vi "Read_Write_Trav_Config.vi"(1 "Traverse Name":string, 2 "Mode":T1(ring)) -> (0 "Error String":string)   [LabVIEW 2022 SP3]
uses:
  Anemometry/Anemometry Sub Vis/Globals/Constants_global.vi
  DriveConfigGlobal.vi
  Anemometry/Anemometry Sub Vis/Globals/Trav_pos_global.vi
  Serial Link Layer/subVIs/Serial_Logging_Global.vi
  <vilib>/Instr/_visa.llb/VISA Find Search Mode.ctl
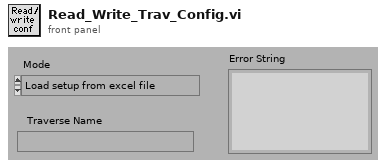
[diagram p1: front panel]
types:
  T1 = enum16{"Load setup from excel file", "Save setup to excel file"}
  T2 = typedef "DriveProperties.ctl" = cluster{"Channel Name":string, "Vel. Default":sgl, "Acc. Default":sgl, "Vel. Max":sgl, "Vel. Min":sgl, "Acc. Max":sgl, "Acc. Min":sgl, "Pulses/unit":sgl, "Address":u8, "Pulse Offset":i32, "Pos Tolerance":sgl, "Pulses/rev":sgl, "Backlash/Eng units":sgl, "Current Pos":sgl, "Ch Status":enum16{"Active", "Offline", "Simulate"}, "Port Name":string, "Axis Transform mode":string, "Metadata Ch Name":string, "Type":string, "De Power Motor":enum16{"TRUE", "FALSE"}, "ConfigString":string}
  T3 = typedef "VISA Find Search Mode.ctl" = u32
  T4 = typedef "Port_Params.ctl" = cluster{"Name":string, "flow control etc.":cluster{"input XON/XOFF":bool, "input HW Handshake":bool, "input alt HW HShk":bool, "output XON/XOFF":bool, "output HW Handshake":bool, "output alt HW HShk":bool, "XOFF byte ":u8, "XON byte":u8, "parity err byte":u16}, "buffer size":u16, "baud rate":u32, "data bits":u16, "stop bits":enum16{"1 bit", "1.5 bits", "2 bits"}, "parity":enum16{"no parity", "odd parity", "even parity", "mark parity", "space parity"}}
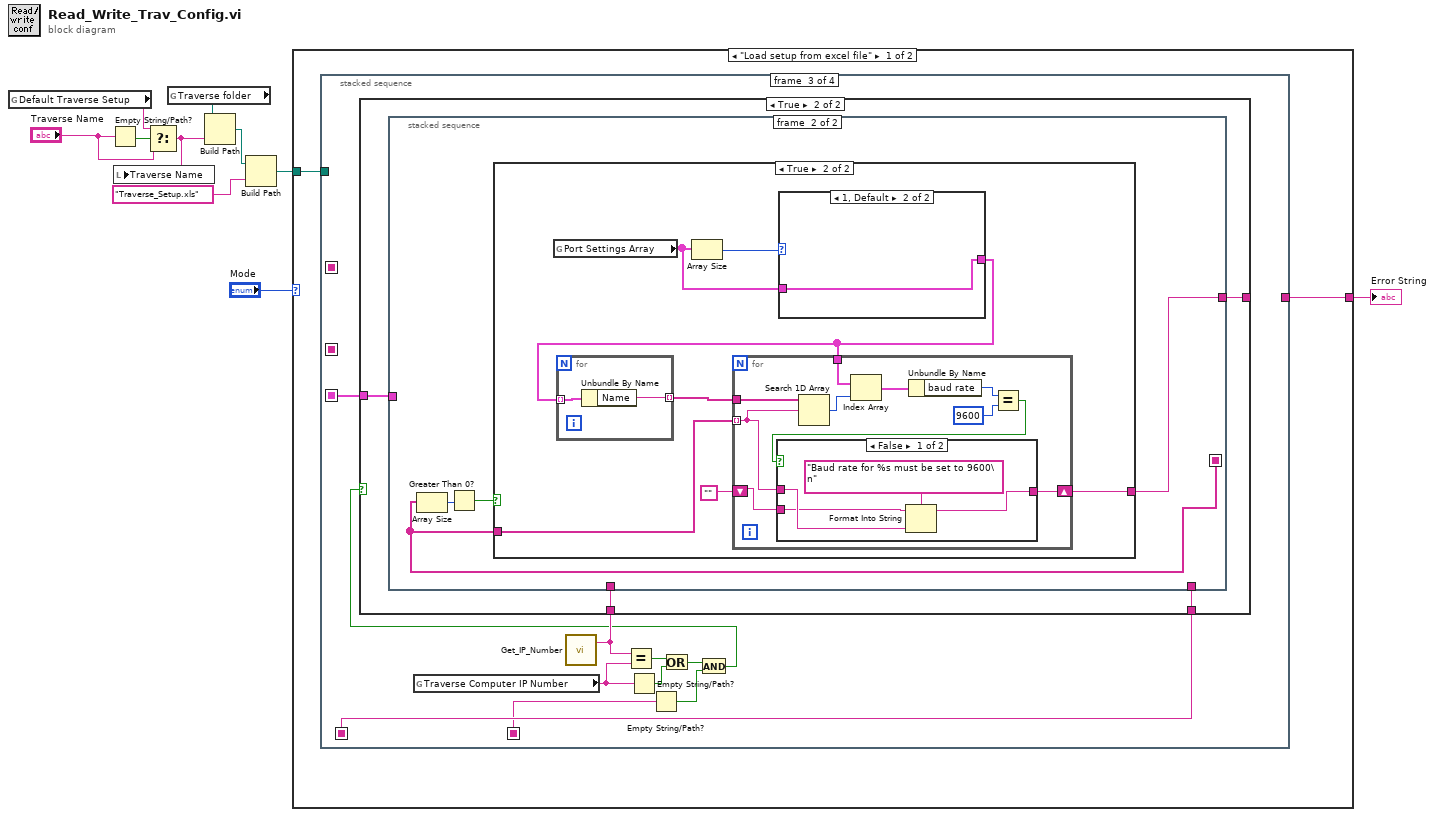
[diagram p0: block diagram]
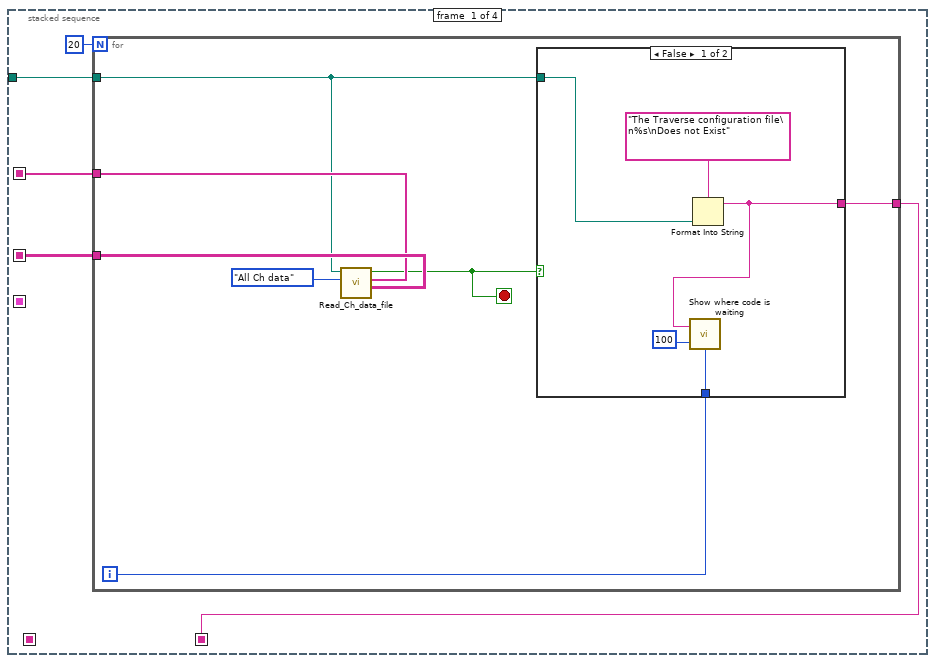
[diagram p2: hidden frame]
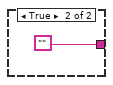
[diagram p3: hidden frame]
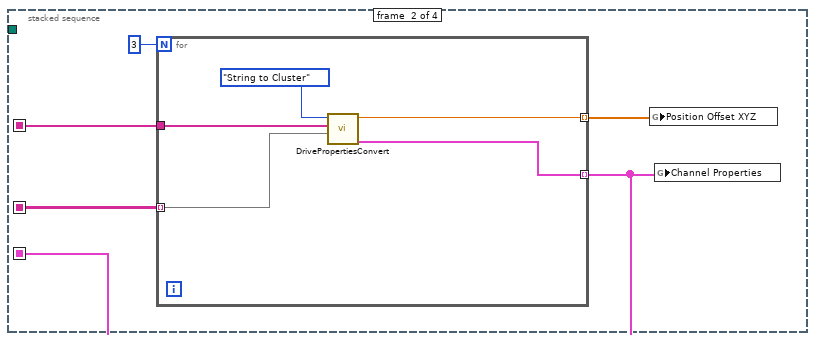
[diagram p4: hidden frame]
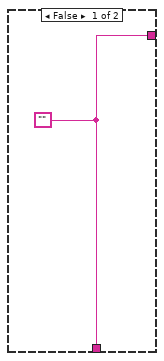
[diagram p5: hidden frame]
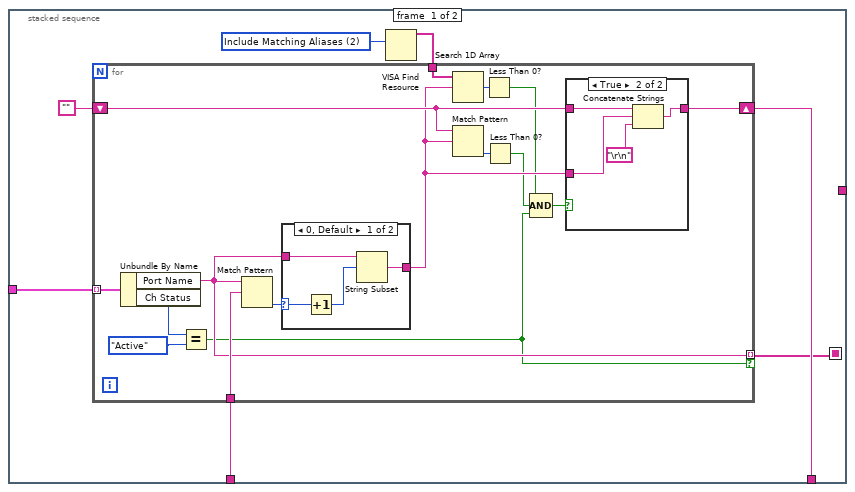
[diagram p6: hidden frame]
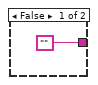
[diagram p9: hidden frame]
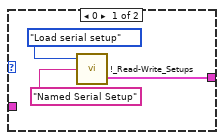
[diagram p11: hidden frame]
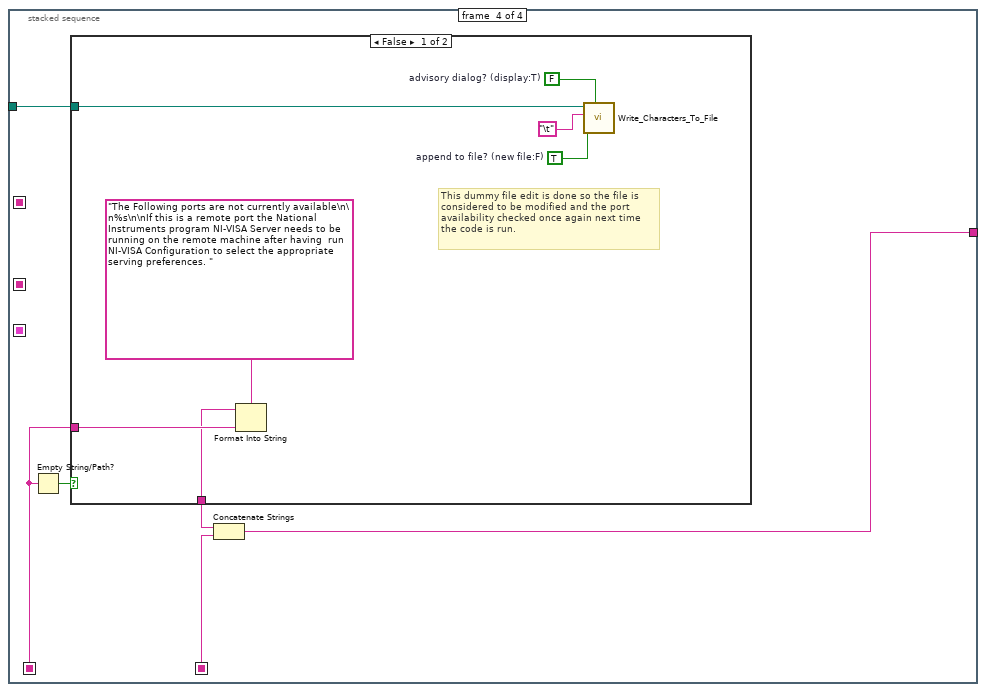
[diagram p12: hidden frame]
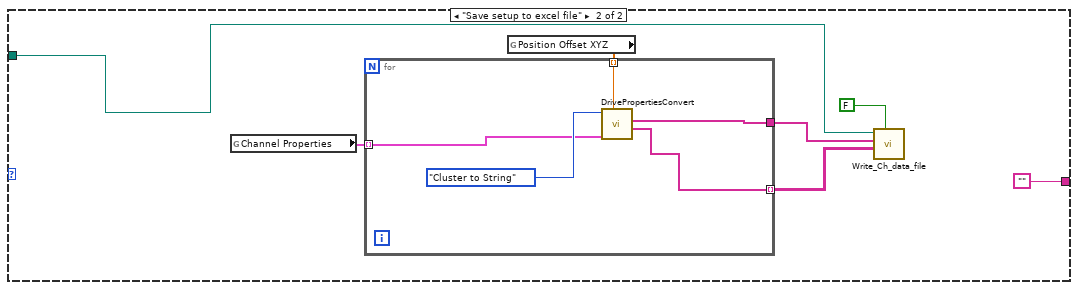
[diagram p14: hidden frame]
diagram:
  n1 = global read "Trav_pos_global.vi" "Default Traverse Setup"() -> (w5:string)
  n2 = Empty String/Path?(string/path="Traverse Name") -> (empty?=w6:bool)
  n3 = Select(t=w5, s=w6, f="Traverse Name") -> (s? t:f=w2:string)
  n4 = local write "Traverse Name"(w2) -> ()
  n5 = global read "Constants_global.vi" "Traverse folder"() -> (w8:path)
  n6 = Build Path(base path=w8, name or relative path=w2) -> (appended path=w7:path)
  n7 = Build Path(base path=w7, name or relative path="Traverse_Setup.xls" ("Substring")) -> (appended path=w9:path)
  n8 = case shown="\"Load setup from excel file\"" "Mode" {
    tunnel: w9 -> [w12 w142]
    tunnel: [w11 ""] -> w1
    frame "Load setup from excel file" {
      n9 = stacked-sequence {
        seq-local: [w17 _ _ _] -> [_ w34 _ _]
        seq-local: [w16 _ _ _] -> [_ w35 _ _]
        seq-local: [_ w33 _ _] -> [_ _ w50 _]
        seq-local: [_ _ w49 _] -> [_ _ _ w126]
        seq-local: [w13 _ _ _] -> [_ _ w41 w123]
        tunnel: w12 -> [w15 _ _ w125]
        tunnel: [_ _ _ w122] -> w11
        frame #0 {
          n10 = for {
            N: 20 -> [_]
            tunnel: [w23] -> w17
            tunnel: [w22] -> w16
            tunnel: w15 -> [w21]
            tunnel: [w20] -> w13
            i -> [w18]
            stop <- w19 stop-if-true
            n11 = call "Read_Ch_data_file.vi"("Output"=enum16{"All Ch data", "The last few rows"}."All Ch data", "Filename"=w21) -> ("Channel Values"=w23:string[][], "Merged Channels"=w22:string[], "exists?"=w19:bool)  [unwired: 3 in, 2 out]
            n12 = case shown="False" w19 {
              tunnel: w21 -> [w29 _]
              tunnel: [w26 ""] -> w20
              tunnel: w18 -> [w25 _]
              frame False {
                n13 = Format Into String(format string="The Traverse configuration file\n%s\nDoes not Exist" ("Format String"), w29) -> (resulting string=w26:string)  [unwired: 2 in, 1 out]
                n14 = call "Show where code is waiting.vi"("Loop index"=w25, "Wait (ms)"=u32 100 ("milliseconds to wait"), "Message"=w26) -> ()  [unwired: 1 in]
              }
              frame True {
              }
            }
          }
        }
        frame #1 {
          n15 = for {
            N: 3 -> [_]
            tunnel: w35 -> [w39]
            tunnel: w34 -> [w38] mode=indexing
            tunnel: [w36] -> w33 mode=indexing
            tunnel: [w37] -> w32 mode=indexing
            n16 = call "DrivePropertiesConvert.vi"("String in"=w38, "Ch names In"=w39, "Mode"=enum16{"Cluster to String", "String to Cluster"}."String to Cluster") -> ("Channel Properties Out"=w36:T2, "Position Offset Out"=w37:dbl)  [unwired: 2 in, 2 out]
          }
          n17 = global write "DriveConfigGlobal.vi" "Position Offset XYZ"(w32) -> ()
          n18 = global write "DriveConfigGlobal.vi" "Channel Properties"(w33) -> ()
        }
        frame #2 {
          n19 = global read "Trav_pos_global.vi" "Traverse Computer IP Number"() -> (w47:string)
          n20 = call "Get_IP_Number.vi"() -> ("IP Number"=w48:string)  [unwired: 1 out]
          n21 = Equal?(x=w48, y=w47) -> (x = y?=w45:bool)
          n22 = Empty String/Path?(string/path=w47) -> (empty?=w46:bool)
          n23 = Empty String/Path?(string/path=w41) -> (empty?=w44:bool)
          n24 = Or(x=w45, y=w46) -> (x .or. y?=w43:bool)
          n25 = And(x=w43, y=w44) -> (x .and. y?=w42:bool)
          n26 = case shown="True" w42 {
            tunnel: w50 -> [_ w55]
            tunnel: [w51 w54] -> w49
            tunnel: w48 -> [_ w53]
            tunnel: [w51 w52] -> _
            frame False {
              w51 = ""
            }
            frame True {
              n27 = stacked-sequence {
                seq-local: [w57 _] -> [_ w90]
                tunnel: w55 -> [w62 _]
                tunnel: [w59 _] -> w54
                tunnel: w53 -> [w58 _]
                tunnel: [_ w89] -> w52
                frame #0 {
                  w56 = T3 2 items=["Canonical Names Only"=0, "Aliases Only"=1, "Include Matching Aliases"=2, "Include All Aliases"=4] ("Search Mode")
                  n28 = VISA Find Resource(10:w56) -> (3:w61:string[])  [unwired: 1 in, 3 out]
                  n29 = for {
                    tunnel: w58 -> [w78]
                    tunnel: w62 -> [w76] mode=indexing
                    tunnel: w61 -> [w75]
                    shift-right: [w74] -> w59
                    shift-left: "" -> [w73]
                    tunnel: [w66] -> w57 mode=indexing if=w65
                    n30 = Unbundle By Name(w76) -> ("Port Name"=w66:string, "Ch Status"=w64:enum16{"Active", "Offline", "Simulate"})
                    n31 = Equal?(x=w64, y=enum16{"Active", "Offline", "Simulate"}."Active" ("Channel Properties.Ch Status")) -> (x = y?=w65:bool)
                    n32 = Match Pattern(string=w66, regular expression=w78) -> (offset past match=w77:i32)  [unwired: 4 out]
                    n33 = case shown="0, Default" w77 {
                      selector: w77 -> [w84 _]
                      tunnel: [w85 w88] -> w72
                      tunnel: w66 -> [w86 w88]
                      frame 0, Default {
                        n34 = Increment(x=w84) -> (x+1=w87:i32)
                        n35 = String Subset(string=w86, offset (0)=w87) -> (substring=w85:string)  [unwired: 1 out]
                      }
                      frame -1 {
                      }
                    }
                    n36 = Search 1D Array(1D array=w75, element=w72) -> (index of element=w71:i32)  [unwired: 1 out]
                    n37 = Match Pattern(string=w73, regular expression=w72) -> (offset past match=w70:i32)  [unwired: 4 out]
                    n38 = Less Than 0?(x=w71) -> (x < 0?=w63:bool)
                    n39 = Less Than 0?(x=w70) -> (x < 0?=w68:bool)
                    n40 = Compound Arithmetic op=AND(w63, w68, w65) -> (w69:bool)
                    n41 = case shown="True" w69 {
                      tunnel: w73 -> [w79 w83]
                      tunnel: [w79 w82] -> w74
                      tunnel: w72 -> [_ w81]
                      frame False {
                      }
                      frame True {
                        n42 = Concatenate Strings(w83, w81, "\r\n") -> (w82:string)
                      }
                    }
                  }
                }
                frame #1 {
                  n43 = Array Size(array=w90) -> (size(s)=w92:i32)
                  n44 = Greater Than 0?(x=w92) -> (x > 0?=w91:bool)
                  n45 = case shown="True" w91 {
                    tunnel: w90 -> [_ w98]
                    tunnel: ["" w94] -> w89
                    frame False {
                    }
                    frame True {
                      n46 = global read "Serial_Logging_Global.vi" "Port Settings Array"() -> (w95:T4[])
                      n47 = Array Size(array=w95) -> (size(s)=w100:i32)
                      n48 = case shown="1, Default" w100 {
                        tunnel: [w118 w121] -> w97
                        tunnel: w95 -> [_ w121]
                        frame 0 {
                          n49 = call "!_Read-Write_Setups.vi"("Setup Name"="Named Serial Setup", "Mode"=enum16{"Load serial setup", "Save serial setup"}."Load serial setup") -> ("Port Settings Array Out"=w118:T4[])  [unwired: 1 in, 1 out]
                        }
                        frame 1, Default {
                        }
                      }
                      n50 = for {
                        tunnel: w97 -> [w117] mode=indexing
                        tunnel: [w116] -> w99 mode=indexing
                        n51 = Unbundle By Name(w117) -> ("Name"=w116:string)
                      }
                      n52 = for {
                        tunnel: w99 -> [w110]
                        tunnel: w98 -> [w103] mode=indexing
                        tunnel: w97 -> [w108]
                        shift-right: [w102] -> w94
                        shift-left: "" -> [w101]
                        n53 = Search 1D Array(1D array=w110, element=w103) -> (index of element=w109:i32)  [unwired: 1 in]
                        n54 = Index Array(array=w108, index=w109) -> (element=w107:T4)
                        n55 = Unbundle By Name(w107) -> ("baud rate"=w105:u32)
                        n56 = Equal?(x=w105, y=u32 9600 ("baud rate")) -> (x = y?=w104:bool)
                        n57 = case shown="False" w104 {
                          tunnel: w103 -> [w114 _]
                          tunnel: [w112 w115] -> w102
                          tunnel: w101 -> [w111 w115]
                          frame False {
                            n58 = Format Into String(format string="Baud rate for %s must be set to 9600\n", initial string=w111, w114) -> (resulting string=w112:string)  [unwired: 1 in, 1 out]
                          }
                          frame True {
                          }
                        }
                      }
                    }
                  }
                }
              }
            }
          }
        }
        frame #3 {
          n59 = Empty String/Path?(string/path=w126) -> (empty?=w127:bool)
          n60 = case shown="False" w127 {
            tunnel: w126 -> [w134 w135]
            tunnel: w125 -> [w133 _]
            tunnel: [w128 w135] -> w124
            frame False {
              w129 = FALSE  # advisory dialog? (display:T)
              w130 = TRUE  # append to file? (new file:F)
              # "This dummy file edit is done so the file is \nconsidered to be modified and the port \navailability checked once again next time\nthe code is run."
              n61 = Format Into String(format string="The Following ports are not currently available\n\n%s\n\nIf this is a remote port the National Instruments program NI-VISA Server needs to be running on the remote machine after having  run NI-VISA Configuration to select the appropriate serving preferences. ", w134) -> (resulting string=w128:string)  [unwired: 2 in, 1 out]
              n62 = call "Write_Characters_To_File.vi"("file path (dialog if empty)"=w133, "advisory dialog? (display:T)"=w129, "character string"="\t", "append to file? (new file:F)"=w130) -> ()  [unwired: 1 in, 4 out]
            }
            frame True {
            }
          }
          n63 = Concatenate Strings(w124, w123) -> (w122:string)
        }
      }
    }
    frame "Save setup to excel file" {
      n64 = global read "DriveConfigGlobal.vi" "Channel Properties"() -> (w140:T2[])
      n65 = global read "DriveConfigGlobal.vi" "Position Offset XYZ"() -> (w139:dbl[])
      n66 = for {
        tunnel: w140 -> [w145] mode=indexing
        tunnel: [w144] -> w137
        tunnel: [w143] -> w136 mode=indexing
        tunnel: w139 -> [w146] mode=indexing
        n67 = call "DrivePropertiesConvert.vi"("Position Offset In"=w146, "Channel Properties In"=w145, "Mode"=enum16{"Cluster to String", "String to Cluster"}."Cluster to String") -> ("String Values"=w143:string[], "Ch names"=w144:string[])  [unwired: 2 in, 2 out]
      }
      n68 = call "Write_Ch_data_file.vi"("exists?"=FALSE, "Channel Values"=w136, "Channel names"=w137, "Filename"=w142) -> ()  [unwired: 3 in, 5 out]
    }
  }
  "Error String" <- w1
